vi "Transfer Group.Errors.Return Timeout.vi"(7 "error source vi name":string, 8 "error in (no error)":errorcluster, 10 "expected iteration":u64=1, 11 "Transfer Group in":refnum<class "Transfer Group.lvclass">) -> (0 "error out":errorcluster, 3 "Transfer Group out":refnum<class "Transfer Group.lvclass">)   [LabVIEW 2017, in "DSF Core.lvlib" / "Transfer Group.lvclass"]
uses:
  Transfer Group.lvclass
  Transfer Group.lvclass/Transfer Group.ctl
  Shared/Constants/Engine Library Name.vi
  <vilib>/NI/Memory Manager/VIs/New Error Cluster Constant (512B).vi
  <vilib>/NI/Memory Manager/VIs/Source.Write.Scalar.Base10 (I32).vi
  <vilib>/NI/Memory Manager/VIs/Source.Write.Scalar.Base10 (U64).vi
  DSF Core.lvlib
  <vilib>/NI/Memory Manager/Static Error Handling.lvlib
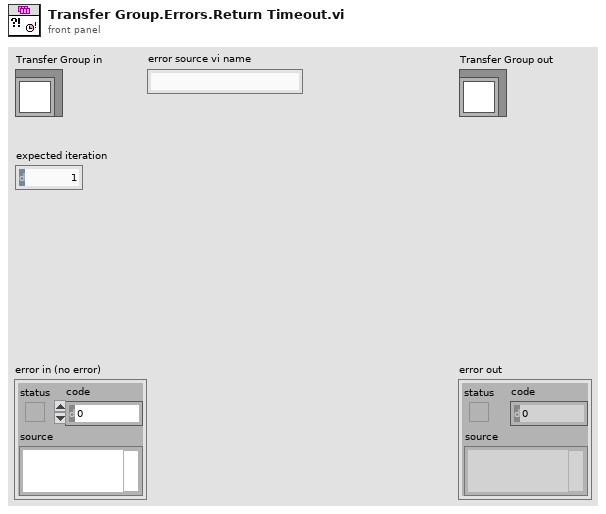
[diagram p1: front panel]
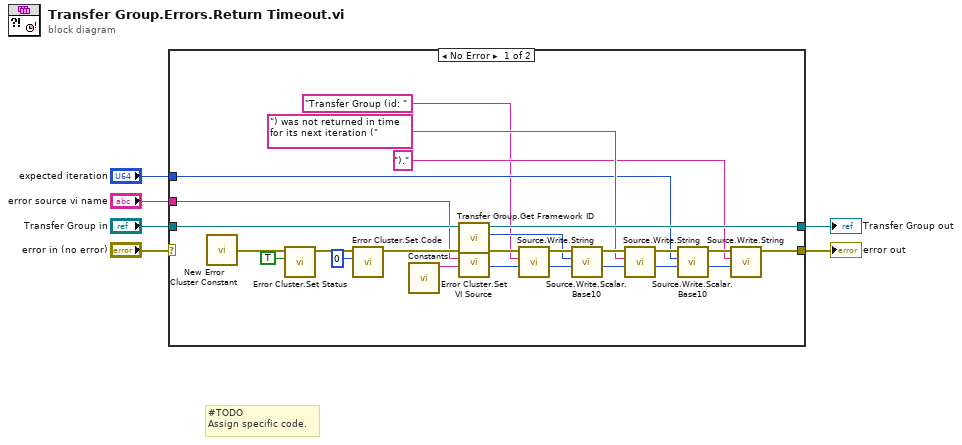
[diagram p0: block diagram]
diagram:
  # "#TODO\nAssign specific code."
  n1 = case shown="No Error" "error in (no error)" {
    selector: "error in (no error)" -> [_ w32]
    tunnel: [w12 w32] -> w5
    tunnel: [w24 w33] -> w4
    tunnel: "Transfer Group in" -> [w25 w33]
    tunnel: "error source vi name" -> [w17 _]
    tunnel: "expected iteration" -> [w14 _]
    frame No Error {
      n2 = call-poly <vilib>:"New Error Cluster Constant.vi"() -> ("error out"=w31:errorcluster)  [unwired: 1 in]
      n3 = call <vilib>:"Error Cluster.Set Status.vi"("status (T)"=TRUE, "error in"=w31) -> ("error out"=w30:errorcluster)  [unwired: 9 in]
      n4 = call <vilib>:"Error Cluster.Set Code.vi"("code"=0, "error in"=w30) -> ("error out"=w28:errorcluster)  [unwired: 9 in]
      n5 = call-poly "Constants.vi"() -> ("Engine Library Name"=w27:string)  [unwired: 11 in]
      n6 = call "Transfer Group.Get Framework ID.vi"("Transfer Group in"=w25) -> ("framework id"=w21:i32, "Transfer Group out"=w24:refnum<class "Transfer Group.lvclass">)  [unwired: 9 in]
      n7 = call <vilib>:"Error Cluster.Set VI Source.vi"("library name (\"\")"=w27, "vi name"=w17, "error in"=w28) -> ("new offset"=w8:i32, "error out"=w26:errorcluster)  [unwired: 7 in]
      n8 = call <vilib>:"Source.Write.String.vi"("offset"=w8, "string"="Transfer Group (id: ", "error in"=w26) -> ("new offset"=w22:i32, "error out"=w23:errorcluster)  [unwired: 7 in]
      n9 = call-poly <vilib>:"Source.Write.Scalar.Base10.vi"("offset"=w22, "value"=w21, "error in"=w23) -> ("new offset"=w19:i32, "error out"=w20:errorcluster)  [unwired: 7 in]
      n10 = call <vilib>:"Source.Write.String.vi"("offset"=w19, "string"=") was not returned in time for its next iteration (", "error in"=w20) -> ("new offset"=w15:i32, "error out"=w16:errorcluster)  [unwired: 7 in]
      n11 = call-poly <vilib>:"Source.Write.Scalar.Base10.vi"("offset"=w15, "value"=w14, "error in"=w16) -> ("new offset"=w11:i32, "error out"=w13:errorcluster)  [unwired: 7 in]
      n12 = call <vilib>:"Source.Write.String.vi"("offset"=w11, "string"=").", "error in"=w13) -> ("error out"=w12:errorcluster)  [unwired: 7 in, 1 out]
    }
    frame Error {
      # "Incoming error. Pass through."
    }
  }
  "error out" <- w5
  "Transfer Group out" <- w4
